vi "Manual not Manual.vi"(9 "Current Angle":dbl) -> (2 "Angle Power":dbl)   [LabVIEW 2017]
uses:
  Robot Global Data.vi
  <vilib>/addons/control/pid/pid.llb/PID (DBL).vi
  <vilib>/addons/control/pid/NI_PID_pid.lvlib
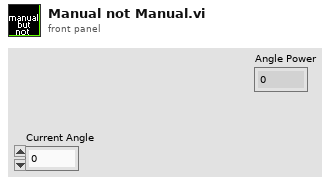
[diagram p1: front panel]
types:
  T1 = typedef "Intake Command Cluster.ctl" = cluster{"Intake Mode":T2, "Intake States":T3, "Manual Roller Power":dbl, "Manual Close?":bool, "Manual Lift Power":dbl, "Override Lift?":bool, "Override Angle":dbl, "Manual Dropmid":bool, "Manual Shoot Angle":bool}
  T2 = typedef "Intake Mode.ctl" = enum16{"Auto", "Semi Auto", "Manual"}
  T3 = typedef "Intake States.ctl" = enum16{"Zero", "Override Angle", "Idle", "Drop Mid", "Drop Low", "Outtake", "Intake"}
  T4 = typedef "Dashboard Control Data.ctl" = cluster{"Drivetrain Settings Cluster":T5, "Intake Presets":T7, "Elevator Settings Cluster":T8, "Drivetrain Encoder Values":T10, "Auton Chooser":T11, "Auton Presets":cluster{"Start Position":dbl}, "Elevator Encoder Values":T12, "Pressure M":dbl, "Pressure B":dbl, "Zero All?":bool, "Enable Vision":bool}
  T5 = typedef "Drivetrain Settings Cluster.ctl" = cluster{"Gyro Steer PID Gains":T6, "Distance Drive PID Gains":T6, "Drive Tolerance":dbl, "Gyro Tolerance":dbl, "Gyro Output":dbl, "Distance Output":dbl, "Y Power Multiplier":dbl, "Turn Power Multiplier":dbl, "Creep Rate":dbl, "Encoder Reset":bool, "DT Mode Modifier":enum16{"None, Default", "Cube", "Square"}, "Left Encoder Tick Constant":dbl, "Right Encoder Tick Constant":dbl, "Shift Speed":dbl, "Zero Gyro":bool, "Y min":dbl, "Y max":dbl, "X min":dbl, "X max":dbl, "Finish Velocity":dbl, "Anti-tip peRcEnT":dbl}
  T6 = typedef "PID Gains Cluster.ctl" = cluster{"Proportional Gain":dbl, "Integral Time":dbl, "Derivative Time":dbl}
  T7 = typedef "Intake Presets.ctl" = cluster{"Idle Angle":dbl, "Mid Angle":dbl, "Low Angle":dbl, "Outtake Power":dbl, "Intake Power":dbl, "Unstuck":dbl, "Angle Tolerance":dbl, "Max Angle":dbl, "Max Current":dbl, "Current Trip Time":dbl, "Reset Encoder?":bool, "Encoder Scale":dbl, "PID gains":cluster{"proportional gain (Kc)":dbl, "integral time (Ti, min)":dbl, "derivative time (Td, min)":dbl}, "output range":cluster{"output high":dbl, "output low":dbl}, "IR Constant Pull Rate":dbl, "Shoot Angle":dbl}
  T8 = typedef "Elevator Settings Cluster.ctl" = cluster{"Ground Height":dbl, "Switch Height":dbl, "Scale High Height ":dbl, "Scale Low Height":dbl, "Elevator PID Gains":T9, "Elevator Tolerance":dbl, "Reset Encoders":bool, "Encoder Scale":dbl, "Max Height":dbl, "Mid Height":dbl, "output range":cluster{"output high":dbl, "output low":dbl}, "Upper Slow Down Tolerance":dbl, "Tick Constant":dbl, "Tip Constant":dbl, "Slow Down Multiplier":dbl, "Almost Tip Constant":dbl, "Bottom Trip Offset":dbl, "Lower Slow Down Tolerance":dbl}
  T9 = typedef "PID Gains.ctl" = cluster{"proportional gain (Kc)":dbl, "integral time (Ti, min)":dbl, "derivative time (Td, min)":dbl}
  T10 = typedef "DT Encoder Values.ctl" = cluster{"Left Encoder":cluster{"Distance":dbl, "Speed":dbl, "Tick":dbl}, "Right Encoder":cluster{"Distance":dbl, "Speed":dbl, "Tick":dbl}}
  T11 = typedef "Auton Chooser.ctl" = cluster{"Left":bool, "Center":bool, "Right":bool, "Scale":bool, "Both":bool, "Switch":bool, "Test":bool, "No Script":bool, "Drive PID":bool, "Elevator PID":bool, "Gyro PID":bool}
  T12 = typedef "Elevator Encoder Values.ctl" = cluster{"Encoder Values":cluster{"Distance":dbl, "Speed":dbl, "Tick":dbl}}
  T13 = cluster{"proportional gain (Kc)":dbl, "integral time (Ti, min)":dbl, "derivative time (Td, min)":dbl}
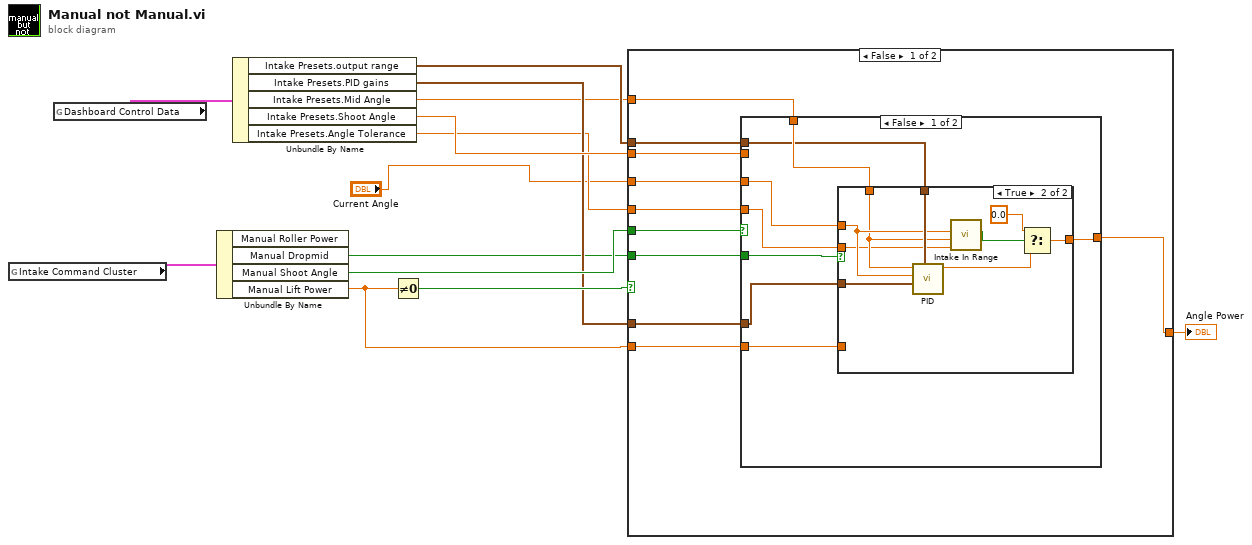
[diagram p0: block diagram]
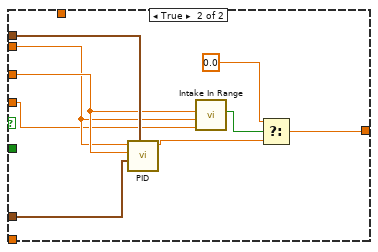
[diagram p3: hidden frame]
diagram:
  n1 = global read "Robot Global Data.vi" "Intake Command Cluster"() -> (w13:T1)
  n2 = global read "Robot Global Data.vi" "Dashboard Control Data"() -> (w8:T4)
  n3 = Unbundle By Name(w13) -> ("Manual Dropmid"=w3:bool, "Manual Shoot Angle"=w9:bool, "Manual Lift Power"=w11:dbl)  [unwired: 1 out]
  n4 = Unbundle By Name(w8) -> ("Intake Presets.output range"=w6:cluster{"output high":dbl, "output low":dbl}, "Intake Presets.PID gains"=w5:T13, "Intake Presets.Mid Angle"=w2:dbl, "Intake Presets.Shoot Angle"=w7:dbl, "Intake Presets.Angle Tolerance"=w4:dbl)
  n5 = Not Equal To 0?(x=w11) -> (x != 0?=w12:bool)
  n6 = case shown="False" w12 {
    tunnel: w11 -> [w14 w51]
    tunnel: [w18 w51] -> w10
    tunnel: w9 -> [w23 _]
    tunnel: w7 -> [w22 _]
    tunnel: "Current Angle" -> [w21 _]
    tunnel: w6 -> [w15 _]
    tunnel: w5 -> [w20 _]
    tunnel: w4 -> [w19 _]
    tunnel: w3 -> [w17 _]
    tunnel: w2 -> [w16 _]
    frame False {
      n7 = case shown="False" w23 {
        tunnel: w22 -> [_ w47]
        tunnel: w21 -> [w29 w48]
        tunnel: w20 -> [w27 w49]
        tunnel: w19 -> [w26 w46]
        tunnel: [w25 w42] -> w18
        tunnel: w17 -> [w31 _]
        tunnel: w16 -> [w30 _]
        tunnel: w15 -> [w28 w50]
        tunnel: w14 -> [w24 _]
        frame False {
          n8 = case shown="True" w31 {
            tunnel: w30 -> [_ w37]
            tunnel: w29 -> [_ w38]
            tunnel: w28 -> [_ w41]
            tunnel: w27 -> [_ w40]
            tunnel: w26 -> [_ w36]
            tunnel: [w32 w33] -> w25
            tunnel: w24 -> [w32 _]
            frame False {
            }
            frame True {
              n9 = call-poly <vilib>:"PID.vi"("output range"=w41, "PID gains"=w40, "process variable"=w38, "setpoint"=w37) -> ("output"=w35:dbl)  [unwired: 6 in, 1 out]
              n10 = call "Intake In Range.vi"("Angle Tolerance"=w36, "Target Height"=w37, "Actual Height"=w38) -> ("In Range?"=w39:bool)  [unwired: 8 in]
              n11 = Select(t=0.0, s=w39, f=w35) -> (s? t:f=w33:dbl)
            }
          }
        }
        frame True {
          n12 = call-poly <vilib>:"PID.vi"("output range"=w50, "PID gains"=w49, "process variable"=w48, "setpoint"=w47) -> ("output"=w43:dbl)  [unwired: 6 in, 1 out]
          n13 = call "Intake In Range.vi"("Angle Tolerance"=w46, "Target Height"=w47, "Actual Height"=w48) -> ("In Range?"=w45:bool)  [unwired: 8 in]
          n14 = Select(t=0.0, s=w45, f=w43) -> (s? t:f=w42:dbl)
        }
      }
    }
    frame True {
    }
  }
  "Angle Power" <- w10
